vi "CRYGet MultiListBox Click State.vi"(10 "Coords":T1, 11 "MultiList Box Ref In":refnum<vi>) -> (0 "Column":i32, 1 "Row":i32, 2 "State":bool, 3 "MultiList Box Ref Out":refnum<vi>)   [LabVIEW 2013]
uses:
  <vilib>/Utility/miscctls.llb/LVPoint32TypeDef.ctl
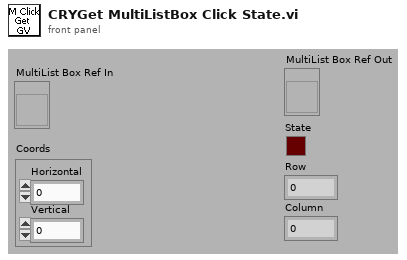
[diagram p1: front panel]
types:
  T1 = typedef "LVPoint32TypeDef.ctl" = cluster{"Horizontal":i32, "Vertical":i32}
  T2 = typedef "LVRowAndColumnTypeDef.ctl" = cluster{"Row":i32, "Column":i32}
  T3 = typedef "LVBoundsTypeDef.ctl" = cluster{"Width":u32, "Height":u32}
  T4 = typedef "LVPositionTypeDef.ctl" = cluster{"Left":i32, "Top":i32}
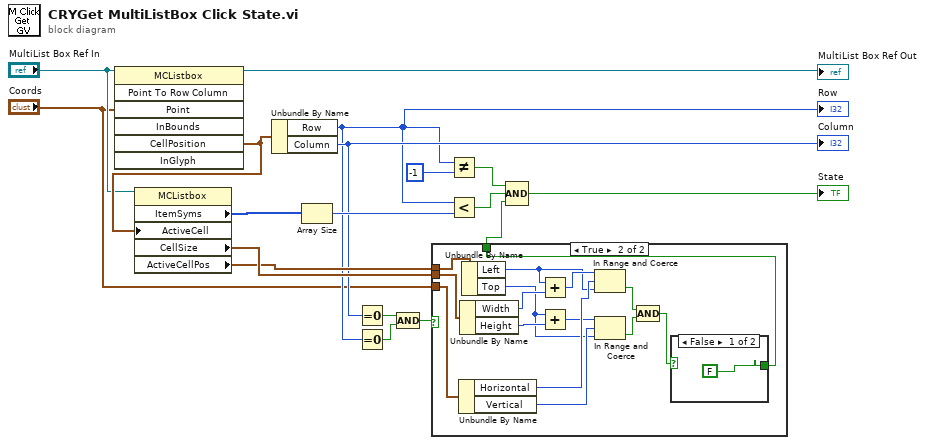
[diagram p0: block diagram]
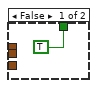
[diagram p2: hidden frame]
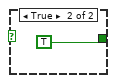
[diagram p3: hidden frame]
diagram:
  n1 = invoke on="Invoke Node" class="MCListbox" method="Point To Row Column"(reference="MultiList Box Ref In", "Point"="Coords") -> (reference out=→"MultiList Box Ref Out":refnum<vi>, "CellPosition"=w6:T2)  [unwired: 5 in, 5 out]
  n2 = property on="Property Node" class="MCListbox"(reference="MultiList Box Ref In", "ActiveCell"=w6) -> ("ItemSyms"=w7:i32[], "CellSize"=w10:T3, "ActiveCellPos"=w9:T4)  [unwired: 1 in, 2 out]
  n3 = Unbundle By Name(w6) -> ("Row"=w4:i32, "Column"=w5:i32)
  "Row" <- w4
  "Column" <- w5
  n4 = Array Size(array=w7) -> (size(s)=w16:i32)
  n5 = Equal To 0?(x=w5) -> (x = 0?=w13:bool)
  n6 = Equal To 0?(x=w4) -> (x = 0?=w12:bool)
  n7 = Compound Arithmetic op=AND(w13, w12) -> (w11:bool)
  n8 = case shown="True" w11 {
    tunnel: w9 -> [_ w33]
    tunnel: "Coords" -> [_ w34]
    tunnel: w10 -> [_ w32]
    tunnel: [TRUE w20] -> w8
    frame False {
    }
    frame True {
      n9 = Unbundle By Name(w34) -> ("Horizontal"=w25:i32, "Vertical"=w29:i32)
      n10 = Unbundle By Name(w32) -> ("Width"=w31:u32, "Height"=w30:u32)
      n11 = Unbundle By Name(w33) -> ("Left"=w23:i32, "Top"=w21:i32)
      n12 = Add(x=w23, y=w31) -> (x+y=w24:u32)
      n13 = Add(x=w21, y=w30) -> (x+y=w22:u32)
      n14 = In Range and Coerce(upper limit=w24, x=w25, lower limit=w23) -> (In Range?=w28:bool)  [unwired: 1 out]
      n15 = In Range and Coerce(upper limit=w22, x=w29, lower limit=w21) -> (In Range?=w27:bool)  [unwired: 1 out]
      n16 = Compound Arithmetic op=AND(w28, w27) -> (w26:bool)
      n17 = case shown="False" w26 {
        tunnel: [FALSE TRUE] -> w20
        frame False {
        }
        frame True {
        }
      }
    }
  }
  n18 = Not Equal?(x=w4, y=-1) -> (x != y?=w14:bool)
  n19 = Less?(x=w4, y=w16) -> (x < y?=w15:bool)
  n20 = Compound Arithmetic op=AND(w14, w15, w8) -> (→"State":bool)
